vi "libpropPage_1Library_Settings.vi"(8 "error in (no error)":errorcluster) -> ()   [LabVIEW 2020]
doc: "This is the general settings page for a project library."
uses:
  <resource>/Framework/Providers/VILibrary/LIBUIP_messages.ctl
  <vilib>/Utility/error.llb/DialogType.ctl
  <resource>/Framework/Providers/VILibrary/LIBUIP_global_LibInfo.vi
  <resource>/Framework/Providers/VILibrary/libFrame_PageVIData.ctl
  <resource>/Framework/Providers/VILibrary/libFrame_LockEvent.ctl
  <resource>/dialog/PreferencesDialog/optionsFrame_EventData1.ctl
panel:
  in  "set text icon on vis":bool
  in  "Save version":string(combo)="Default"
  in  "set text icon":bool
  in  "sourceOnly":bool
  out "Source Version":string
  in  "apply icon":bool
  in  "Fix":u16
  in  "Build":u16
  in  "Minor":u16
  in  "Major":u16
  in  "Icon":picture
  in  "edit icon":bool
  in  "B & W":picture
  in  "Default Palette":u16(ring) items=["None"]
  out "Library Path":path
  in  "stop event in":refnum<user-event>
  in  "page events in":refnum<user-event>
  in  "page synch rendezvous":T1
  in  "Page VI Data":T2
  # "VI Icon Template"
  # "Version Number"
  # "."
  # "."
  # "."
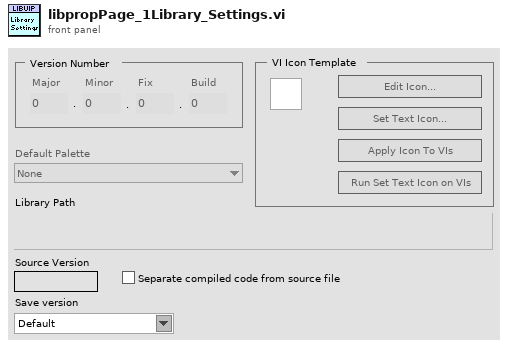
[diagram p1: front panel]
types:
  T1 = typedef "Rendezvous RefNum" = refnum<k1>
  T2 = typedef "libFrame_PageVIData.ctl" = cluster{"page VIs paths":path[], "Library Refnum":refnum<vi>, "Initial Lock State":enum32{"invalid lock state", "Not Locked", "Locked (No Password)", "Password-protected"}, "pwd in cache":bool}
  T3 = typedef "LIBUIP_messages.ctl" = enum16{"Initialize", "Handle User Events", "Update Panel", "Redraw Tree"}
  T4 = enum32{"invalid lock state", "Not Locked", "Locked (No Password)", "Password-protected"}
  T5 = typedef "LIBUIP_library_info.ctl" = cluster{"Path":path, "Version":cluster{"major":u16, "minor":u16, "fix":u16, "build":u16}, "B&W Icon":picture, "256 Icon":picture, "Lock State":enum32{"invalid lock state", "Not Locked", "Locked (No Password)", "Password-protected"}, "pwd cached":bool, "Default Menu":string, "Synchronize mnu":bool, "source Version":string, "sourceOnly":bool, "Save Version":string}
  T6 = enum8{"Enabled", "Disabled", "Disabled and Grayed Out"}
  T7 = typedef "imagedata.ctl" = cluster{"image type":i32, "image depth":i32, "image":u8[], "mask":u8[], "colors":u32[], "Rectangle":cluster{"left":i16, "top":i16, "right":i16, "bottom":i16}}
  T8 = cluster{"Major":u16, "Minor":u16, "Fix":u16, "Build":u16}
  T9 = typedef "DialogType.ctl" = u16
  T10 = cluster{"Lock State":enum32{"invalid lock state", "Not Locked", "Locked (No Password)", "Password-protected"}, "pwd cached":bool, "String":string}
  T11 = cluster{"major":u16, "minor":u16, "fix":u16, "build":u16}
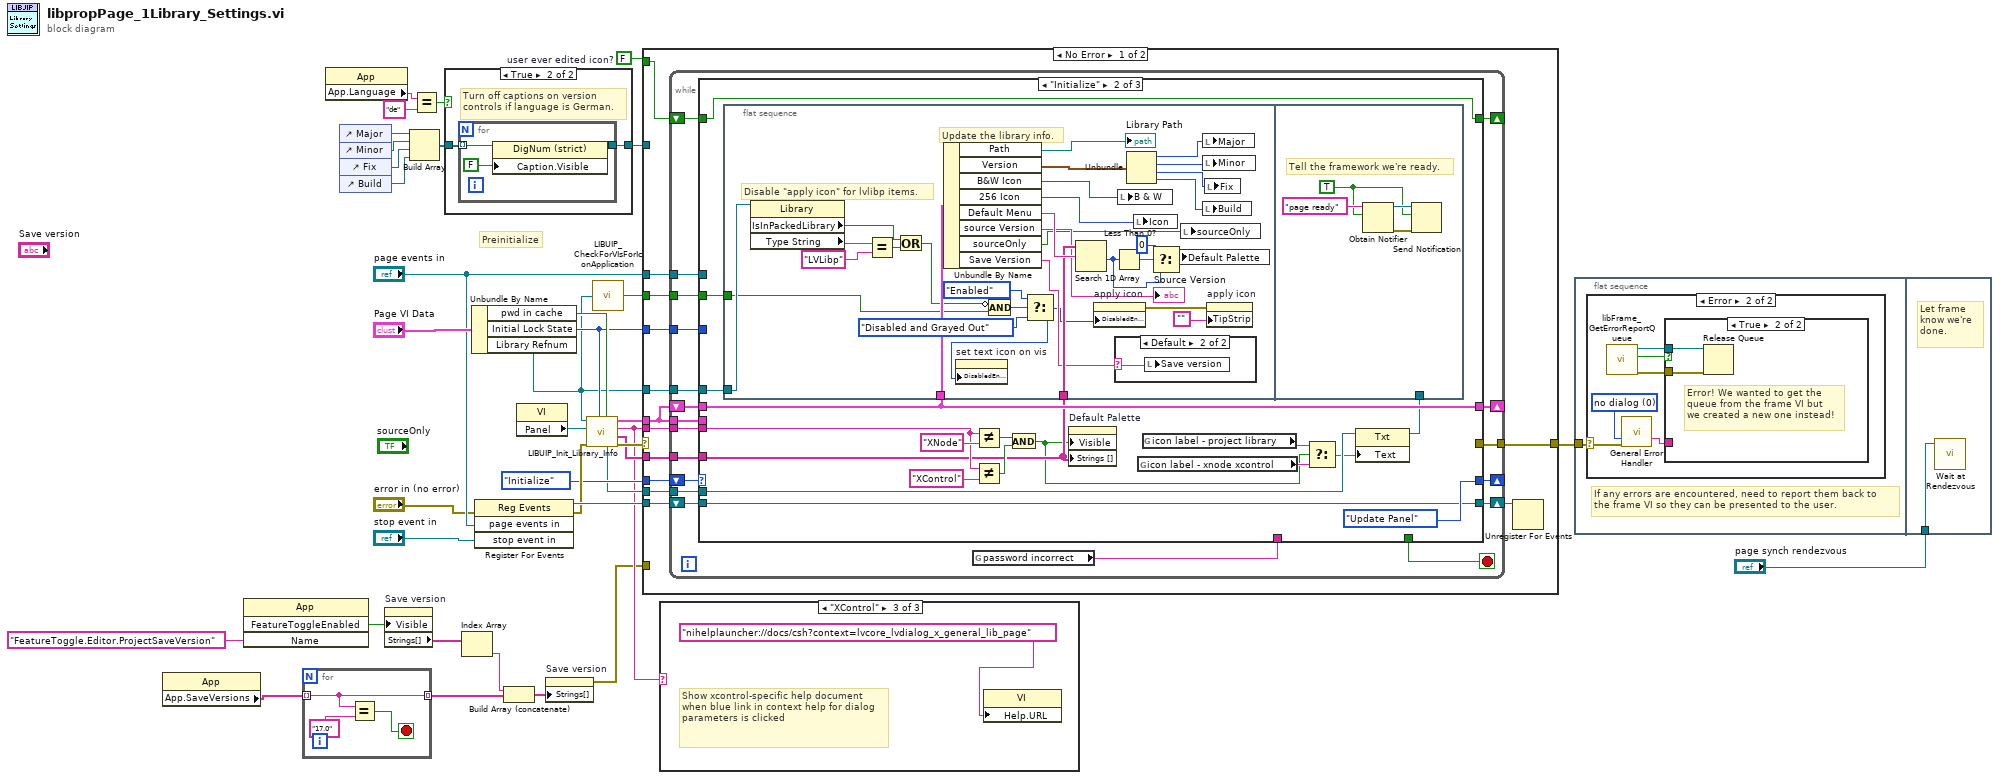
[diagram p0: block diagram]
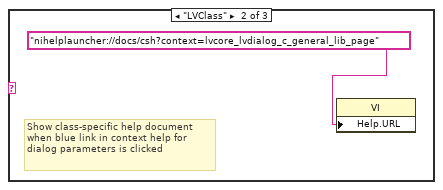
[diagram p3: hidden frame]
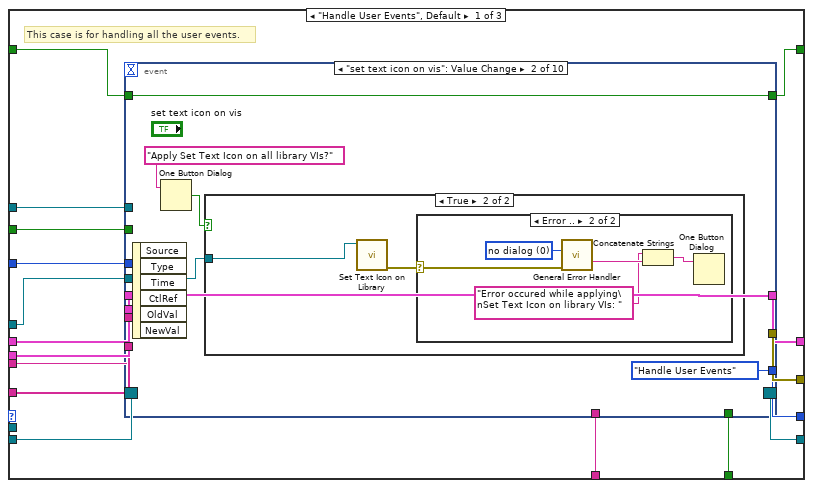
[diagram p5: hidden frame]
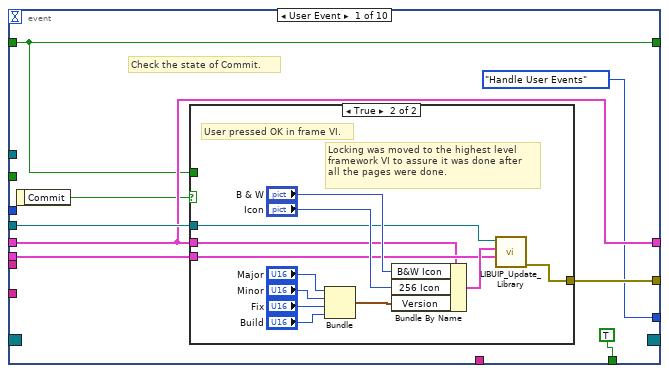
[diagram p6: hidden frame]
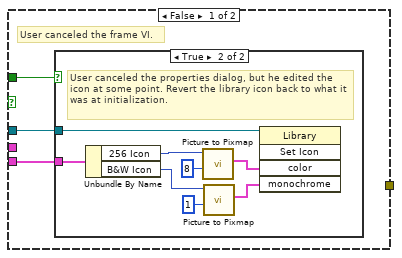
[diagram p7: hidden frame]
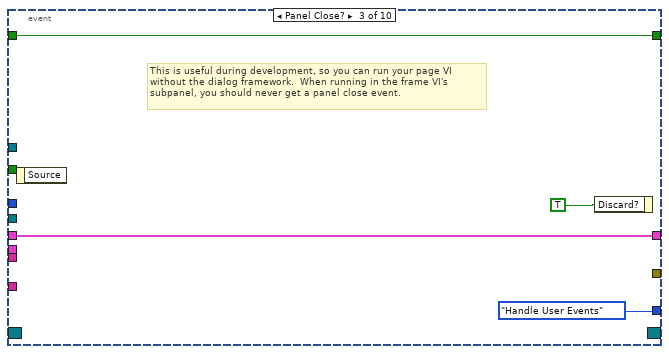
[diagram p11: hidden frame]
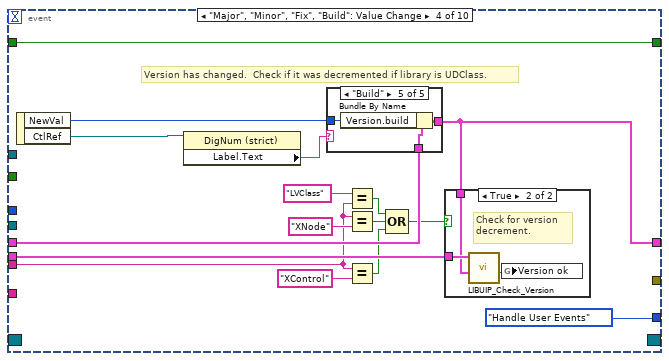
[diagram p12: hidden frame]
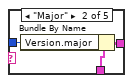
[diagram p14: hidden frame]
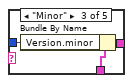
[diagram p15: hidden frame]
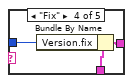
[diagram p16: hidden frame]
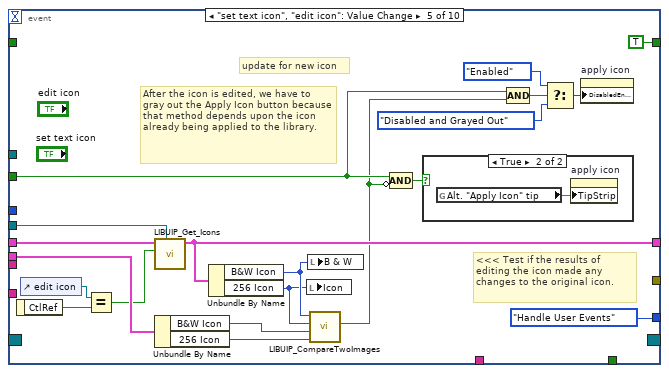
[diagram p18: hidden frame]
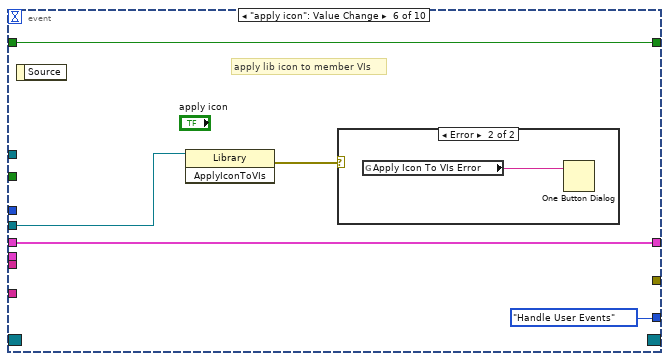
[diagram p20: hidden frame]
diagram:
  w10 = FALSE  # user ever edited icon?
  # "Preinitialize"
  n1 = property class="App"() -> ("App.SaveVersions"=w2:string[])  [unwired: 2 in, 2 out]
  n2 = invoke class="App" method="FeatureToggleEnabled"("Name"="FeatureToggle.Editor.ProjectSaveVersion" ("TokenName")) -> ("FeatureToggleEnabled"=w5:bool)  [unwired: 3 in, 3 out]
  n3 = for {
    tunnel: [w40] -> w3 mode=indexing
    tunnel: w2 -> [w40] mode=indexing
    stop <- w38 stop-if-true
    n4 = Equal?(x=w40, y="17.0") -> (x = y?=w38:bool)
  }
  n5 = property class="App"() -> ("App.Language"=w21:string)  [unwired: 2 in, 2 out]
  n6 = control-ref of="Major"() -> (w19:refnum<vi>)
  n7 = control-ref of="Minor"() -> (w18:refnum<vi>)
  n8 = control-ref of="Fix"() -> (w17:refnum<vi>)
  n9 = control-ref of="Build"() -> (w16:refnum<vi>)
  n10 = property on="Save version" class="CmbBox"("Visible"=w5) -> ("Strings[]"=w6:string[])  [unwired: 2 in, 2 out]
  n11 = Build Array(w19, w18, w17, w16) -> (w14:refnum<vi>[])
  n12 = Equal?(x=w21, y="de") -> (x = y?=w15:bool)
  n13 = case shown="True" w15 {
    tunnel: w14 -> [_ w42]
    tunnel: [_ w41] -> w13
    frame False {
    }
    frame True {
      # "Turn off captions on version\ncontrols if language is German."
      n14 = for {
        tunnel: w42 -> [w44] mode=indexing
        tunnel: [w43] -> w41
        n15 = property on="Property Node" class="DigNum (strict)"(reference=w44, "Caption.Visible"=FALSE) -> (reference out=w43:refnum<vi>)  [unwired: 1 in, 1 out]
      }
    }
  }
  n16 = Index Array(array=w6) -> (element=w7:string)  [unwired: 1 in]
  n17 = Unbundle By Name("Page VI Data") -> ("pwd in cache"=w23:bool, "Initial Lock State"=w22:T4, "Library Refnum"=w12:refnum<vi>)
  n18 = register-events(error in="error in (no error)", "page events in", "stop event in") -> (reference out=w35:refnum<event-registration>, error out=w33:errorcluster)  [unwired: 1 in]
  n19 = Build Array (concatenate)(w7, w3) -> (w8:string[])
  n20 = property class="VI"() -> ("Panel"=w24:refnum<vi>)  [unwired: 2 in, 2 out]
  n21 = property on="Save version" class="CmbBox"("Strings[]"=w8) -> (error out=w1:errorcluster)  [unwired: 2 in, 1 out]
  n22 = call <resource>:"LIBUIP_Init_Library_Info.vi"("pwd cached"=w23, "Lock State"=w22, "error in (no error)"=w33, "Pnl Refnum"=w24, "Library Refnum"=w12) -> ("error out"=w28:errorcluster, "Menu Files"=w27:string[], "Library Type"=w9:string, "Library Info"=w32:T5, "Txt Refnum"=w25:refnum<vi>)  [unwired: 2 out]
  n23 = call <resource>:"LIBUIP_CheckForVIsForIconApplication.vi"("Library Refnum"=w12) -> ("Has VIs?"=w11:bool)
  n24 = case shown="No Error" w28 {
    selector: w28 -> [_ w313]
    tunnel: w12 -> [w58 _]
    tunnel: w35 -> [w56 _]
    tunnel: [w55 w313] -> w34
    tunnel: w32 -> [w54 _]
    tunnel: LIBUIP_messages."Initialize" ("element") -> [w53 _]
    tunnel: w27 -> [w52 _]
    tunnel: "page events in" -> [w51 _]
    tunnel: w9 -> [w50 _]
    tunnel: w25 -> [w49 _]
    tunnel: w22 -> [w48 _]
    tunnel: w13 -> [_ _]
    tunnel: w11 -> [w47 _]
    tunnel: w10 -> [w46 _]
    tunnel: w1 -> [_ _]
    frame No Error {
      n25 = while {
        tunnel: [w77] -> w55
        shift-right: [w76] -> _
        shift-left: w54 -> [w75]
        tunnel: w58 -> [w73]
        tunnel: w51 -> [w74]
        tunnel: w54 -> [w72]
        shift-right: [w71] -> w57
        shift-left: w56 -> [w70]
        shift-right: [w68] -> _
        shift-left: w53 -> [w69]
        tunnel: w52 -> [w67]
        tunnel: w50 -> [w64]
        tunnel: w49 -> [w63]
        tunnel: w48 -> [w62]
        tunnel: w47 -> [w61]
        shift-right: [w59] -> _
        shift-left: w46 -> [w60]
        stop <- w65 stop-if-true
        n26 = global read "LIBUIP_global_LibInfo.vi" "password incorrect"() -> (w66:string)
        n27 = case shown="\"Initialize\"" w69 {
          tunnel: [w94 _ _] -> w77
          tunnel: [w91 w256 w312] -> w76
          tunnel: w73 -> [w89 w240 _]
          tunnel: w75 -> [w93 w256 w312]
          tunnel: w70 -> [w92 w254 w306]
          tunnel: w74 -> [w90 _ _]
          tunnel: w72 -> [w88 _ _]
          tunnel: w66 -> [w87 _ _]
          tunnel: [w86 w254 w306] -> w71
          tunnel: [w85 LIBUIP_messages."Update Panel" ("element") LIBUIP_messages."Handle User Events" ("element")] -> w68
          tunnel: [w84 _ _] -> w65
          tunnel: w67 -> [w83 w248 _]
          tunnel: w64 -> [w82 w251 _]
          tunnel: w63 -> [_ w243 _]
          tunnel: w62 -> [w81 _ _]
          tunnel: w61 -> [w80 w241 _]
          tunnel: w60 -> [w79 w239 w294]
          tunnel: [w78 w239 w294] -> w59
          frame "Handle User Events", Default {
            # "This case is for handling all the user events."
            n28 = event shown="[1] \"set text icon on vis\": Value Change" {
              selector: w92 -> [_ _ _ _ _ _ _ _ _ _]
              dyn-events: [_ _ _ _ _ _ _ _ _ _] -> w86
              timeout: _ -> [_ _ _ _ _ _ _ _ _ _]
              tunnel: [w99 _ _ _ _ _ _ _ _ _] -> w94
              tunnel: w93 -> [w100 w127 w141 w157 w194 w199 w209 w220 w225 w233]
              tunnel: [w100 w127 w141 w153 w193 w199 w216 w219 w224 w232] -> w91
              tunnel: w90 -> [_ _ _ _ _ _ w208 _ _ _]
              tunnel: w89 -> [w102 w128 _ _ w191 w197 _ _ _ _]
              tunnel: w88 -> [w101 _ _ w154 w190 _ _ _ _ _]
              tunnel: w87 -> [_ _ _ _ _ _ _ _ _ _]
              tunnel: [LIBUIP_messages."Handle User Events" ("element") LIBUIP_messages."Handle User Events" ("element") LIBUIP_messages."Handle User Events" ("element") LIBUIP_messages."Handle User Events" ("element") LIBUIP_messages."Handle User Events" ("element") LIBUIP_messages."Handle User Events" ("element") LIBUIP_messages."Update Panel" ("element") LIBUIP_messages."Handle User Events" ("element") LIBUIP_messages."Handle User Events" ("element") LIBUIP_messages."Update Panel" ("element")] -> w85
              tunnel: [TRUE _ _ _ _ _ _ _ _ _] -> w84
              tunnel: w83 -> [_ _ _ _ _ _ w215 _ _ w235]
              tunnel: w82 -> [_ _ _ w144 _ _ _ _ _ _]
              tunnel: w81 -> [_ _ _ _ _ _ _ _ _ _]
              tunnel: w80 -> [_ _ _ _ w184 _ _ _ _ _]
              tunnel: w79 -> [w96 w131 w139 w143 _ w196 w202 w217 w222 w227]
              tunnel: [w96 w131 w139 w143 TRUE ("user ever edited icon?") w196 w202 w217 w222 w227] -> w78
              event User Event {
                # "Check the state of Commit."
                n29 = event-data() -> ("Commit"=w95:bool)  [unwired: 1 out]
                n30 = case shown="True" w95 {
                  tunnel: w100 -> [_ w115]
                  tunnel: w102 -> [w104 w114]
                  tunnel: [_ w117] -> w99
                  tunnel: w101 -> [w103 w116]
                  tunnel: w96 -> [w105 _]
                  frame False {
                    # "User canceled the frame VI."
                    n31 = case shown="True" w105 {
                      tunnel: w104 -> [_ w112]
                      tunnel: w103 -> [_ w113]
                      frame False {
                        # "User never edited the icon"
                      }
                      frame True {
                        # "User canceled the properties dialog, but he edited the icon at some point. Revert the library icon back to what it was at initialization."
                        n32 = Unbundle By Name(w113) -> ("256 Icon"=w111:picture, "B&W Icon"=w109:picture)
                        n33 = call <vilib>:"Picture to Pixmap.vi"("depth"=8, "picture"=w111) -> ("image data"=w110:T7)  [unwired: 8 in, 1 out]
                        n34 = call <vilib>:"Picture to Pixmap.vi"("depth"=1, "picture"=w109) -> ("image data"=w108:T7)  [unwired: 8 in, 1 out]
                        n35 = invoke class="Library" method="Set Icon"(reference=w112, "color"=w110, "monochrome"=w108) -> ()  [unwired: 2 in, 5 out]
                      }
                    }
                  }
                  frame True {
                    # "Locking was moved to the highest level \nframework VI to assure it was done after\nall the pages were done."
                    # "User pressed OK in frame VI."
                    n36 = Bundle("Major"="Major", "Minor"="Minor", "Fix"="Fix", "Build"="Build") -> (w119:T8)  [unwired: 1 out]
                    n37 = Bundle By Name(cluster=w115, "B&W Icon"="B & W", "256 Icon"="Icon", "Version"=w119) -> (w118:T5)
                    n38 = call <resource>:"LIBUIP_Update_Library.vi"("Library Info Initial"=w116, "Library Info"=w118, "Library Refnum"=w114) -> ("error out"=w117:errorcluster)  [unwired: 1 in, 7 out]
                  }
                }
              }
              event "set text icon on vis": Value Change {
                n39 = event-data() -> ()  [unwired: 7 out]
                n40 = One Button Dialog(message="Apply Set Text Icon on all library VIs?") -> (true=w130:bool)  [unwired: 1 in]
                n41 = case shown="True" w130 {
                  tunnel: w128 -> [_ w132]
                  frame False {
                  }
                  frame True {
                    n42 = call "Set Text Icon on Library.vi"("reference"=w132) -> ("error out"=w133:errorcluster)  [unwired: 10 in]
                    n43 = case shown="Error .." w133 {
                      selector: w133 -> [_ w137]
                      frame No Error {
                      }
                      frame Error {
                        w138 = T9 0 items=["no dialog", "OK message", "continue or stop message", "OK message + warnings", "continue/stop + warnings"] ("type of dialog (OK msg:1)")
                        n44 = call <vilib>:"General Error Handler.vi"("type of dialog (OK msg:1)"=w138, "error in (no error)"=w137) -> ("message"=w136:string)  [unwired: 1 in, 12 out]
                        n45 = Concatenate Strings("Error occured while applying\nSet Text Icon on library VIs: " ("button name (\"OK\")"), w136) -> (w135:string)
                        n46 = One Button Dialog(message=w135) -> ()  [unwired: 1 in, 1 out]
                      }
                    }
                  }
                }
              }
              event Panel Close? {
                # "This is useful during development, so you can run your page VI \nwithout the dialog framework.  When running in the frame VI's \nsubpanel, you should never get a panel close event."
                n47 = event-data() -> ()  [unwired: 2 out]
                n48 = event-data("Discard?"=TRUE) -> ()  [unwired: 1 in, 1 out]
              }
              event "Major", "Minor", "Fix", "Build": Value Change {
                # "Version has changed.  Check if it was decremented if library is UDClass."
                n49 = event-data() -> ("NewVal"=w155:u16, "CtlRef"=w158:refnum<vi>)  [unwired: 1 out]
                n50 = property class="DigNum (strict)"(reference=w158) -> ("Label.Text"=w156:string)  [unwired: 1 in, 2 out]
                n51 = case shown="\"Build\"" w156 {
                  tunnel: w157 -> [w159 w162 w165 w168 w171]
                  tunnel: [w159 w161 w164 w167 w170] -> w153
                  tunnel: w155 -> [_ w160 w163 w166 w169]
                  frame Default {
                  }
                  frame "Major" {
                    n52 = Bundle By Name(cluster=w162, "Version.major"=w160) -> (w161:T5)
                  }
                  frame "Minor" {
                    n53 = Bundle By Name(cluster=w165, "Version.minor"=w163) -> (w164:T5)
                  }
                  frame "Fix" {
                    n54 = Bundle By Name(cluster=w168, "Version.fix"=w166) -> (w167:T5)
                  }
                  frame "Build" {
                    n55 = Bundle By Name(cluster=w171, "Version.build"=w169) -> (w170:T5)
                  }
                }
                n56 = Equal?(x="LVClass", y=w144) -> (x = y?=w149:bool)
                n57 = Equal?(x=w144, y="XNode") -> (x = y?=w146:bool)
                n58 = Equal?(x=w144, y="XControl") -> (x = y?=w145:bool)
                n59 = Compound Arithmetic op=OR(w149, w146, w145) -> (w150:bool)
                n60 = case shown="True" w150 {
                  tunnel: w154 -> [_ w174]
                  tunnel: w153 -> [_ w173]
                  frame False {
                    # "Generic library; \ndo nothing."
                  }
                  frame True {
                    # "Check for version \ndecrement."
                    n61 = call <resource>:"LIBUIP_Check_Version.vi"("Library Info Current"=w173, "Library Info Initial"=w174) -> ("Version ok?"=w172:bool)  [unwired: 7 out]
                    n62 = global write "LIBUIP_global_LibInfo.vi" "Version ok"(w172) -> ()
                  }
                }
              }
              event "set text icon", "edit icon": Value Change {
                # "After the icon is edited, we have to gray out the Apply Icon button because that method depends upon the icon already being applied to the library."
                # "<<< Test if the results of editing the icon made any changes to the original icon."
                # "update for new icon"
                n63 = event-data() -> ("CtlRef"=w177:refnum<vi>)  [unwired: 1 out]
                n64 = control-ref of="edit icon"() -> (w178:refnum<vi>)
                n65 = Equal?(x=w178, y=w177) -> (x = y?=w176:bool)
                n66 = call <resource>:"LIBUIP_Get_Icons.vi"("Library Refnum"=w191, "launch icon editor"=w176, "Library Info"=w194) -> ("Library Info Out"=w193:T5)  [unwired: 1 in, 7 out]
                n67 = Unbundle By Name(w190) -> ("B&W Icon"=w187:picture, "256 Icon"=w186:picture)
                n68 = Unbundle By Name(w193) -> ("B&W Icon"=w189:picture, "256 Icon"=w188:picture)
                n69 = local write "Icon"(w188) -> ()
                n70 = local write "B & W"(w189) -> ()
                n71 = call <resource>:"LIBUIP_CompareTwoImages.vi"("256 Icon 2"=w186, "B&W Icon 2"=w187, "256 Icon 1"=w188, "B&W Icon 1"=w189) -> ("Both Images Match"=w183:bool)  [unwired: 7 in]
                n72 = Compound Arithmetic op=AND(w184, invert w183) -> (w185:bool)
                n73 = case shown="True" w185 {
                  frame False {
                  }
                  frame True {
                    n74 = global read "LIBUIP_global_LibInfo.vi" "Alt. \"Apply Icon\" tip"() -> (w195:string)
                    n75 = property on="apply icon" class="Bool"("TipStrip"=w195) -> ()  [unwired: 2 in, 2 out]
                  }
                }
                n76 = Compound Arithmetic op=AND(w184, w183) -> (w182:bool)
                n77 = Select(t=T6."Enabled" ("Disabled"), s=w182, f=T6."Disabled and Grayed Out" ("Disabled")) -> (s? t:f=w179:T6)
                n78 = property on="apply icon" class="Bool"("DisabledEnum"=w179) -> ()  [unwired: 2 in, 2 out]
              }
              event "apply icon": Value Change {
                # "apply lib icon to member VIs"
                n79 = event-data() -> ()  [unwired: 2 out]
                n80 = invoke class="Library" method="ApplyIconToVIs"(reference=w197) -> (error out=w198:errorcluster)  [unwired: 2 in, 2 out]
                n81 = case shown="Error" w198 {
                  frame No Error {
                  }
                  frame Error {
                    n82 = global read "LIBUIP_global_LibInfo.vi" "Apply Icon To VIs Error"() -> (w201:string)
                    n83 = One Button Dialog(message=w201) -> ()  [unwired: 1 in, 1 out]
                  }
                }
              }
              event "Default Palette": Value Change {
                # "The default menu has changed; fire event so other pages know."
                n84 = event-data() -> ("NewVal"=w214:u16)  [unwired: 1 out]
                n85 = Index Array(array=w215, index=w214) -> (element=w210:string)
                n86 = Equal?(x=w210, y="None") -> (x = y?=w212:bool)
                n87 = Unbundle By Name(w209) -> ("Lock State"=w207:T4, "pwd cached"=w204:bool)
                n88 = Select(t="", s=w212, f=w210) -> (s? t:f=w206:string)
                n89 = Bundle By Name(cluster=w209, "Default Menu"=w206) -> (w216:T5)
                n90 = Bundle("Lock State"=w207, "pwd cached"=w204, "String"=w206) -> (w203:T10)  [unwired: 1 out]
                n91 = Generate User Event(user event=w208, event data cluster=w203) -> ()  [unwired: 2 in, 2 out]
              }
              event "sourceOnly": Value Change {
                n92 = event-data() -> ("NewVal"=w218:bool)  [unwired: 1 out]
                n93 = Bundle By Name(cluster=w220, "sourceOnly"=w218) -> (w219:T5)
              }
              event "Save version": Value Change {
                n94 = event-data() -> ("NewVal"=w223:string)  [unwired: 1 out]
                n95 = Bundle By Name(cluster=w225, "Save Version"=w223) -> (w224:T5)
              }
              event User Event {
                # "The default menu changed in another page VI; update values."
                n96 = event-data() -> ("Default Menu"=w231:string, "Lock State"=w229:T4, "Password Cached"=w228:bool)  [unwired: 1 out]
                n97 = Search 1D Array(1D array=w235, element=w231) -> (index of element=w236:i32)  [unwired: 1 out]
                n98 = Less Than 0?(x=w236) -> (x < 0?=w238:bool)
                n99 = Bundle By Name(cluster=w233, "Default Menu"=w231, "Lock State"=w229, "pwd cached"=w228) -> (w232:T5)
                n100 = Select(t=0, s=w238, f=w236) -> (s? t:f=w234:i32)
                n101 = local write "Default Palette"(w234) -> ()
              }
            }
          }
          frame "Initialize" {
            n102 = flat-sequence {
              tunnel: w256 -> [w279]
              tunnel: w248 -> [w277]
              tunnel: w241 -> [w263]
              tunnel: w240 -> [w268]
              tunnel: w244 -> [_]
              frame #0 {
                # "Disable \"apply icon\" for lvlibp items."
                # "Update the library info."
                n103 = property class="Library"(reference=w268) -> ("IsInPackedLibrary"=w264:bool, "Type String"=w267:string)  [unwired: 1 in, 2 out]
                n104 = Equal?(x=w267, y="LVLibp") -> (x = y?=w265:bool)
                n105 = Or(x=w264, y=w265) -> (x .or. y?=w262:bool)
                n106 = Unbundle By Name(w279) -> ("Path"=→"Library Path":path, "Version"=w285:T11, "B&W Icon"=w286:picture, "256 Icon"=w287:picture, "Default Menu"=w278:string, "source Version"=→"Source Version":string, "sourceOnly"=w259:bool, "Save Version"=w258:string)
                n107 = Compound Arithmetic op=AND(invert w262, w263) -> (w261:bool)
                n108 = Select(t=T6."Enabled" ("Disabled"), s=w261, f=T6."Disabled and Grayed Out" ("Disabled")) -> (s? t:f=w257:T6)
                n109 = property on="set text icon on vis" class="Bool"("DisabledEnum"=w257) -> ()  [unwired: 2 in, 2 out]
                n110 = Search 1D Array(1D array=w277, element=w278) -> (index of element=w274:i32)  [unwired: 1 out]
                n111 = property on="apply icon" class="Bool"("DisabledEnum"=w257) -> (error out=w272:errorcluster)  [unwired: 2 in, 1 out]
                n112 = Less Than 0?(x=w274) -> (x < 0?=w276:bool)
                n113 = case shown="Default" w258 {
                  selector: w258 -> [_ w288]
                  frame "" {
                  }
                  frame Default {
                    n114 = local write "Save version"(w288) -> ()
                  }
                }
                n115 = local write "B & W"(w286) -> ()
                n116 = Unbundle(w285) -> ("major"=w284:u16, "minor"=w283:u16, "fix"=w282:u16, "build"=w281:u16)
                n117 = local write "Icon"(w287) -> ()
                n118 = Select(t=0, s=w276, f=w274) -> (s? t:f=w273:i32)
                n119 = local write "Default Palette"(w273) -> ()
                n120 = local write "sourceOnly"(w259) -> ()
                n121 = local write "Major"(w284) -> ()
                n122 = local write "Minor"(w283) -> ()
                n123 = local write "Build"(w281) -> ()
                n124 = local write "Fix"(w282) -> ()
                n125 = property on="apply icon" class="Bool"(error in=w272, "TipStrip"="") -> ()  [unwired: 1 in, 2 out]
              }
              frame #1 {
                w290 = TRUE
                # "Tell the framework we're ready."
                n126 = Obtain Notifier(name (unnamed)="page ready", notification data type=w290) -> (notifier out=w291:refnum<notifier>, error out=w289:errorcluster)  [unwired: 2 in, 1 out]
                n127 = Send Notification(notification=w290, notifier=w291, error in (no error)=w289) -> ()  [unwired: 2 out]
              }
            }
            n128 = Not Equal?(x=w251, y="XNode") -> (x != y?=w250:bool)
            n129 = Not Equal?(x=w251, y="XControl") -> (x != y?=w249:bool)
            n130 = And(x=w250, y=w249) -> (x .and. y?=w245:bool)
            n131 = property on="Default Palette" class="Ring (strict)"("Visible"=w245, "Strings []"=w248) -> ()  [unwired: 2 in, 2 out]
            n132 = global read "LIBUIP_global_LibInfo.vi" "icon label - xnode xcontrol"() -> (w246:string)
            n133 = global read "LIBUIP_global_LibInfo.vi" "icon label - project library"() -> (w247:string)
            n134 = Select(t=w247, s=w245, f=w246) -> (s? t:f=w242:string)
            n135 = property class="Txt"(reference=w243, "Text"=w242) -> (reference out=w244:refnum<vi>)  [unwired: 1 in, 1 out]
          }
          frame "Update Panel" {
            # "Source Version"
            # "sourceonly"
            # "used to enable/\ndisable the \nTrack Changes\ncheckbox which \nis now hidden."
            # "Enables and disables items as necessary based on the security settings of the Library."
            n136 = Unbundle By Name(w312) -> ("Lock State"=w305:T4, "pwd cached"=w299:bool)
            n137 = control-ref of="Save version"() -> (w293:refnum<vi>)
            n138 = control-ref of="edit icon"() -> (w296:refnum<vi>)
            n139 = control-ref of="set text icon"() -> (w295:refnum<vi>)
            n140 = control-ref of="sourceOnly"() -> (w298:refnum<vi>)
            n141 = control-ref of="Major"() -> (w310:refnum<vi>)
            n142 = control-ref of="Minor"() -> (w309:refnum<vi>)
            n143 = control-ref of="Fix"() -> (w308:refnum<vi>)
            n144 = control-ref of="Build"() -> (w307:refnum<vi>)
            n145 = control-ref of="Source Version"() -> (w297:refnum<vi>)
            n146 = control-ref of="Default Palette"() -> (w300:refnum<vi>)
            n147 = Build Array(w296, w295, w310, w309, w308, w307, w300, w297, w298, w293) -> (w311:refnum<vi>[])
            n148 = Equal?(x=w305, y=T4."Not Locked") -> (x = y?=w302:bool)
            n149 = Or(x=w302, y=w299) -> (x .or. y?=w301:bool)
            n150 = call <resource>:"provcom_MassEnableDisableControls.vi"("References to alter"=w311, "Enable (TRUE)"=w301) -> ()  [unwired: 1 in, 9 out]
          }
        }
      }
      n151 = Unregister For Events(event registration refnum=w57) -> ()  [unwired: 1 in, 1 out]
    }
    frame Error {
      w315 = FALSE
      # "Error occurred; let the framework know that the page had a problem initializing."
      n152 = Obtain Notifier(name (unnamed)="page ready", notification data type=w315) -> (notifier out=w316:refnum<notifier>, error out=w314:errorcluster)  [unwired: 2 in, 1 out]
      n153 = Send Notification(notification=w315, notifier=w316, error in (no error)=w314) -> ()  [unwired: 2 out]
    }
  }
  n154 = case shown="\"XControl\"" w9 {
    frame Default {
    }
    frame "LVClass" {
      # "Show class-specific help document when blue link in context help for dialog parameters is clicked"
      n155 = property class="VI"("Help.URL"="nihelplauncher://docs/csh?context=lvcore_lvdialog_c_general_lib_page") -> ()  [unwired: 2 in, 2 out]
    }
    frame "XControl" {
      # "Show xcontrol-specific help document when blue link in context help for dialog parameters is clicked"
      n156 = property class="VI"("Help.URL"="nihelplauncher://docs/csh?context=lvcore_lvdialog_x_general_lib_page") -> ()  [unwired: 2 in, 2 out]
    }
  }
  n157 = flat-sequence {
    tunnel: w34 -> [w320]
    tunnel: "page synch rendezvous" -> [w335]
    frame #0 {
      # "If any errors are encountered, need to report them back to \nthe frame VI so they can be presented to the user."
      n158 = case shown="Error" w320 {
        selector: w320 -> [_ w323]
        frame No Error {
        }
        frame Error {
          w321 = T9 0 items=["no dialog", "OK message", "continue or stop message", "OK message + warnings", "continue/stop + warnings"] ("type of dialog (OK msg:1)")
          n159 = call <resource>:"libFrame_GetErrorReportQueue.vi"() -> ("error out"=w324:errorcluster, "created new?"=w326:bool, "queue out"=w325:refnum<queue>)  [unwired: 9 out]
          n160 = call <vilib>:"General Error Handler.vi"("type of dialog (OK msg:1)"=w321, "error in (no error)"=w323) -> ("message"=w322:string)  [unwired: 1 in, 12 out]
          n161 = case shown="True" w326 {
            tunnel: w325 -> [w332 w334]
            tunnel: w324 -> [w331 w333]
            tunnel: w322 -> [w329 _]
            frame False {
              n162 = global read "LIBUIP_global_LibInfo.vi" "error msg string"() -> (w327:string)
              n163 = property class="VI"() -> ("Front Panel.Title"=w330:string)  [unwired: 2 in, 2 out]
              n164 = Format Into String(format string=w327, w330, w329) -> (resulting string=w328:string)  [unwired: 2 in, 1 out]
              n165 = Enqueue Element(queue=w332, element=w328, error in (no error)=w331) -> ()  [unwired: 4 out]
            }
            frame True {
              # "Error! We wanted to get the \nqueue from the frame VI but \nwe created a new one instead!"
              n166 = Release Queue(queue=w334, error in (no error)=w333) -> ()  [unwired: 4 out]
            }
          }
        }
      }
    }
    frame #1 {
      # "Let frame \nknow we're \ndone."
      n167 = call <vilib>:"Wait at Rendezvous.vi"("rendezvous"=w335) -> ()  [unwired: 2 in, 5 out]
    }
  }
